vi "Set Argument - Pythonic.vi"(7 "Function Name":string, 8 "Error In":errorcluster, 9 "Pythonic Value":string, 10 "Argument":string, 11 "OPI Ref":refnum<data-value>) -> (0 "Error Out":errorcluster, 3 "OPI Ref":refnum<data-value>)   [LabVIEW 2012, in "OPI.lvclass"]
doc: "Set string argument value for the future function specified by Function Name. The wired value should be provided in valid pythonic syntax.\n\n<b>Important</b> - use this method to translate pythonic tuples and dictionaries.\n\nThe value is transmitted to the PES. This optimizes the speed with which calls can be made, because no data needs to be transmitted at call time."
uses:
  OPI.lvclass
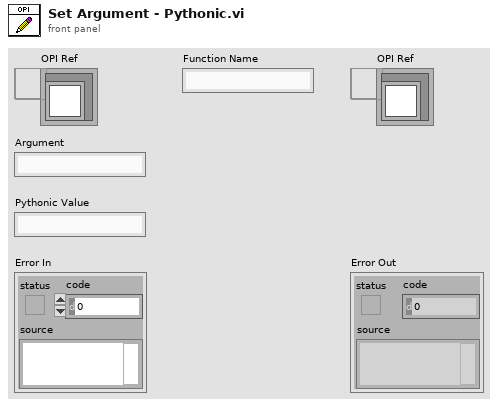
[diagram p1: front panel]
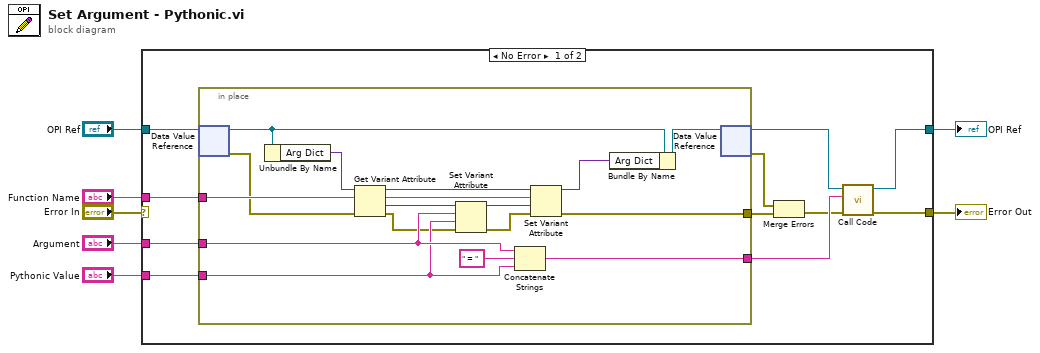
[diagram p0: block diagram]
diagram:
  n1 = case shown="No Error" "Error In" {
    selector: "Error In" -> [_ w35]
    tunnel: "OPI Ref" -> [w18 w36]
    tunnel: "Function Name" -> [w17 _]
    tunnel: [w15 w36] -> w5
    tunnel: "Argument" -> [w14 _]
    tunnel: "Pythonic Value" -> [w13 _]
    tunnel: [w8 w35] -> w1
    frame No Error {
      n2 = in-place {
        in-place-border: w17 -> [w30]
        in-place-border: w14 -> [w25]
        in-place-border: w13 -> [w24]
        in-place-border: [w23] -> w12
        in-place-border: [w19] -> w11
        n3 = in-place-dvr #1(w18) -> (w29:refnum<class "OPI.lvclass">, w22:errorcluster)
        n4 = Unbundle By Name(w29) -> ("Arg Dict"=w34:variant)
        n5 = Get Variant Attribute(Variant=w34, name=w30, error in=w22) -> (duplicate Variant=w32:variant, value=w33:variant, error out=w21:errorcluster)  [unwired: 1 in, 1 out]
        n6 = Set Variant Attribute(Variant=w33, name=w25, value=w24, error in=w21) -> (Variant out=w31:variant, error out=w20:errorcluster)  [unwired: 1 out]
        n7 = Concatenate Strings(w25, " = " ("string"), w24) -> (w23:string)
        n8 = Set Variant Attribute(Variant=w32, name=w30, value=w31, error in=w20) -> (Variant out=w28:variant, error out=w19:errorcluster)  [unwired: 1 out]
        n9 = Bundle By Name(cluster=w29, "Arg Dict"=w28) -> (w27:refnum<class "OPI.lvclass">)
        n10 = in-place-dvr #1(w27) -> (w16:refnum<data-value>, w10:errorcluster)
      }
      n11 = Merge Errors(w10, w11) -> (w9:errorcluster)
      n12 = call "Call Code.vi"("Error In"=w9, "Pythonic Code"=w12, "OPI Ref"=w16) -> ("Error Out"=w8:errorcluster, "OPI Ref"=w15:refnum<data-value>)  [unwired: 7 in]
    }
    frame Error {
    }
  }
  "Error Out" <- w1
  "OPI Ref" <- w5
